vi "Initialize.vi"(8 "error in (no error)":errorcluster, 9 "objects":refnum<class>[](array[class]), 10 "name":string, 11 "Component in":refnum<class "Component.lvclass">) -> (0 "error out":errorcluster, 3 "Component out":refnum<class "Component.lvclass">)   [LabVIEW 2017, in "DSF Core.lvlib" / "Component.lvclass"]
uses:
  Component.lvclass
  Component.lvclass/Component.ctl
  <vilib>/Utility/error.llb/Clear Errors.vi
  Component Configuration/Component Configurations.lvclass
  Component User Interface/Component User Interfaces.lvclass
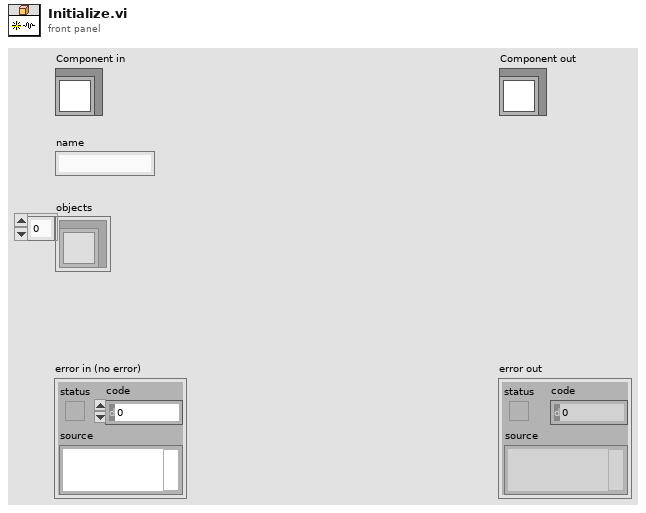
[diagram p1: front panel]
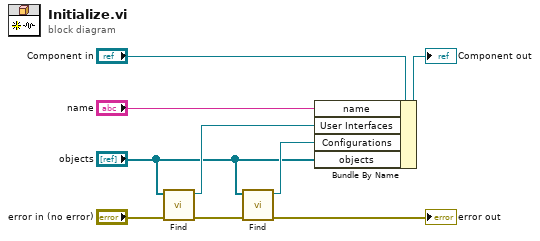
[diagram p0: block diagram]
diagram:
  n1 = call "Find.vi"("error in (no error)"="error in (no error)", "objects"="objects") -> ("error out"=w6:errorcluster, "Component User Interfaces"=w5:refnum<class "Component User Interfaces.lvclass">)  [unwired: 6 in, 2 out]
  n2 = call "Find.vi"("error in (no error)"=w6, "objects"="objects") -> ("error out"=→"error out":errorcluster, "Component Configurations"=w3:refnum<class "Component Configurations.lvclass">)  [unwired: 6 in, 2 out]
  n3 = Bundle By Name(cluster="Component in", "name"="name", "User Interfaces"=w5, "Configurations"=w3, "objects"="objects") -> (→"Component out":refnum<class "Component.lvclass">)
